vi "Handle Signal Density Plot.vi"(7 "State in":T1, 8 "error in (no error)":errorcluster, 10 "Alligned FFT Frame Out":refnum<class "2D Array f32.lvclass">, 11 "Signal Analysis in":refnum<class "Signal Analysis.lvclass">) -> (0 "error out":errorcluster, 2 "Signal Density Plot Available":bool, 3 "Signal Density Plot":refnum<class "2D Array f32.lvclass">, 5 "State out":T1)   [LabVIEW 2020, in "Signal Analysis.lvlib" / "Signal Analysis.lvclass"]
uses:
  Signal Analysis.lvclass
  <vilib>/Natan Biesmans/G2CPU GPU and CPU HPC Toolkit/G2CPU Libraries/Arrays/1DArray/u32/1D Array u32.lvclass
  <vilib>/Natan Biesmans/G2CPU GPU and CPU HPC Toolkit/G2CPU Libraries/Arrays/2DArray/s16/2D Array s16.lvclass
  <vilib>/Natan Biesmans/G2CPU GPU and CPU HPC Toolkit/G2CPU Libraries/Arrays/2DArray/f32/2D Array f32.lvclass
  C:/Program Files/National Instruments/LabVIEW 2025/vi.lib/Natan Biesmans/G2CPU GPU and CPU HPC Toolkit/G2CPU Libraries/Arrays/Array/Array Prototype.lvclass
  Signal Analysis.lvclass/Signal Analysis.ctl
  <vilib>/Natan Biesmans/G2CPU GPU and CPU HPC Toolkit/G2CPU Libraries/Arrays/1DArray/s32/1D Array s32.lvclass
  <vilib>/Natan Biesmans/G2CPU GPU and CPU HPC Toolkit/G2CPU Libraries/Arrays/1DArray/f32/1D Array f32.lvclass
  <vilib>/Natan Biesmans/G2CPU GPU and CPU HPC Toolkit/G2CPU Libraries/Arrays/Array/Array Prototype.lvclass
  <vilib>/Natan Biesmans/G2CPU GPU and CPU HPC Toolkit/G2CPU Libraries/Arrays/DataTypes/I32/s32.lvclass
  <vilib>/Natan Biesmans/G2CPU GPU and CPU HPC Toolkit/G2CPU Libraries/Arrays/1DArray/1D Array Prototype.lvclass
  <vilib>/Natan Biesmans/G2CPU GPU and CPU HPC Toolkit/G2CPU Libraries/Arrays/DataTypes/f32/f32.lvclass
  <vilib>/Natan Biesmans/G2CPU GPU and CPU HPC Toolkit/G2CPU Libraries/Arrays/2DArray/2D Array Prototype.lvclass
  C:/Program Files/National Instruments/LabVIEW 2025/vi.lib/Natan Biesmans/G2CPU GPU and CPU HPC Toolkit/G2CPU Libraries/Arrays/1DArray/1D Array Prototype.lvclass
  C:/Program Files/National Instruments/LabVIEW 2025/vi.lib/Natan Biesmans/G2CPU GPU and CPU HPC Toolkit/G2CPU Libraries/Arrays/1DArray/f32/1D Array f32.lvclass
  C:/Program Files/National Instruments/LabVIEW 2025/vi.lib/Natan Biesmans/G2CPU GPU and CPU HPC Toolkit/G2CPU Libraries/Arrays/DataTypes/f32/f32.lvclass
  d8d0d967-f4c4-454d-b5f2-45f85e871cba.vi
  Program Files/National Instruments/LabVIEW 2025/examples/Natan Biesmans/G2CPU GPU and CPU HPC Toolkit/_Examples/UI Acceleration/Signal Density Plot Config.ctl
  <vilib>/Natan Biesmans/G2CPU GPU and CPU HPC Toolkit/G2CPU Libraries/UI Acceleration/G2CPU Signal Density Plots.lvlib
  0e8233dc-15c9-41dc-9b30-8b63ab7c6b8c.vi
  c5ece696-53a1-4daa-a705-5cda5cc95be4.vi
  <vilib>/Utility/miscctls.llb/LVOffsetAndMultiplierTypeDef.ctl
  Helper Loop State.ctl
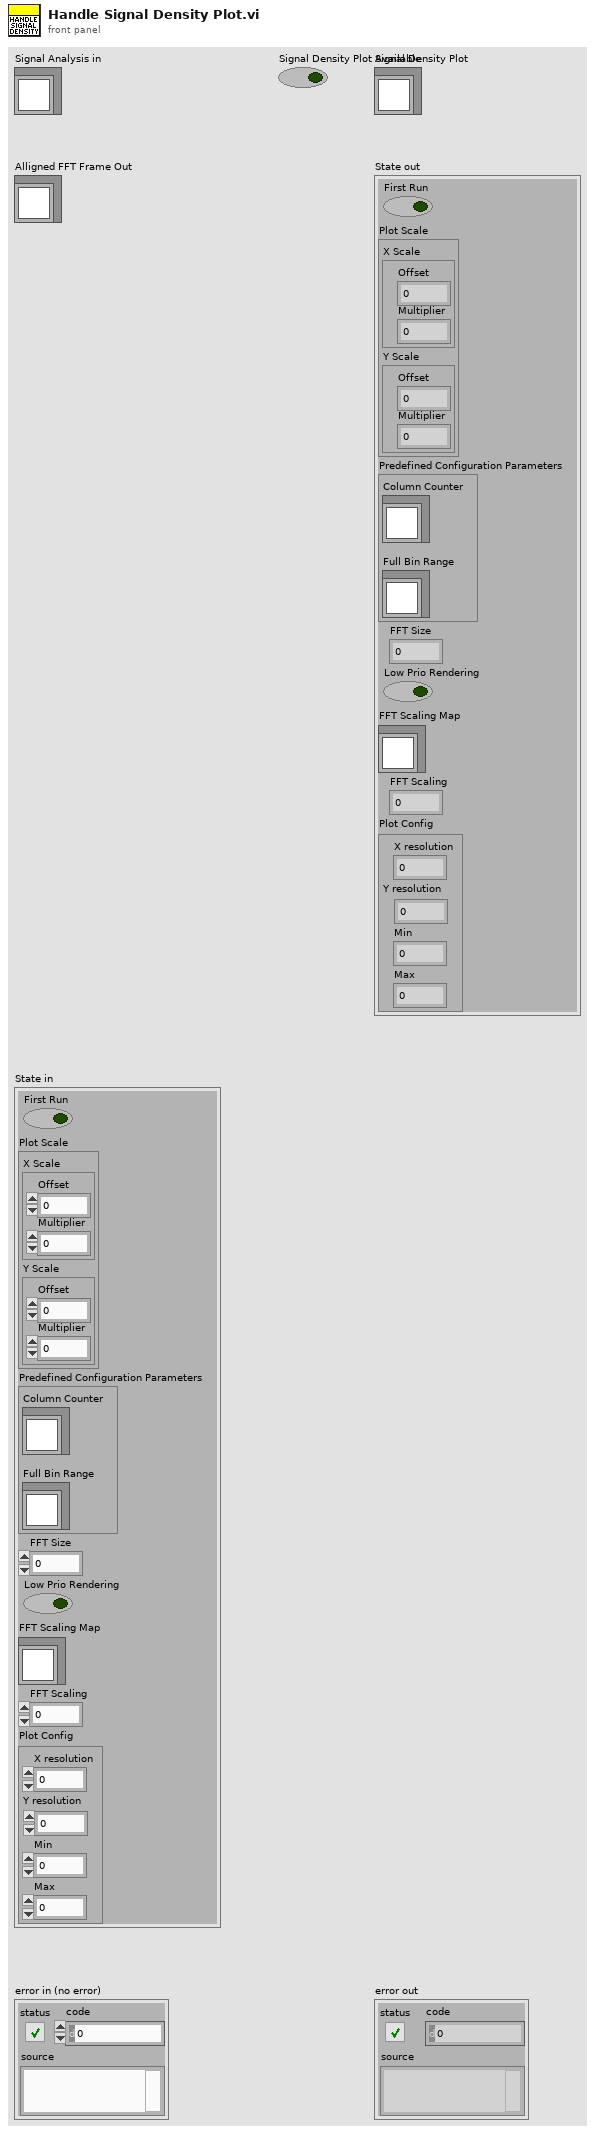
[diagram p1: front panel]
types:
  T1 = typedef "Signal Analysis.lvlib/Signal Analysis.lvclass/Helper Loop State.ctl" = cluster{"First Run":bool, "Plot Scale":cluster{"X Scale":T2, "Y Scale":T2}, "Predefined Configuration Parameters":cluster{"Column Counter":refnum<class "1D Array u32.lvclass">, "Full Bin Range":refnum<class "2D Array s16.lvclass">}, "FFT Size":i32, "Low Prio Rendering":bool, "FFT Scaling Map":refnum<class "1D Array u32.lvclass">, "FFT Scaling":dbl, "Graph Config":T3}
  T2 = typedef "LVOffsetAndMultiplierTypeDef.ctl" = cluster{"Offset":dbl, "Multiplier":dbl}
  T3 = typedef "G2CPU Signal Density Plots.lvlib/Signal Density Plot Config.ctl" = cluster{"X resolution":u64, "Y resolution":u64, "Min":sgl, "Max":sgl}
  T4 = cluster{"Column Counter":refnum<class "1D Array u32.lvclass">, "Full Bin Range":refnum<class "2D Array s16.lvclass">}
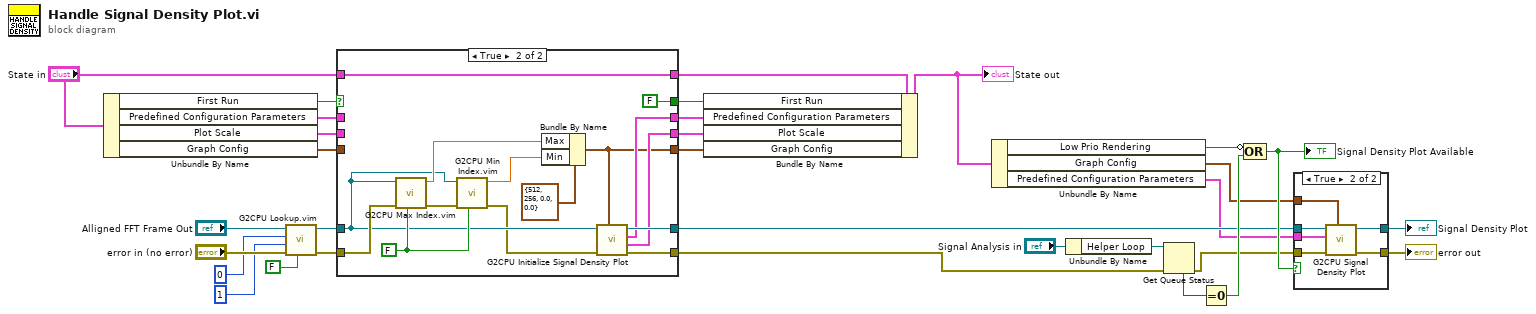
[diagram p0: block diagram]
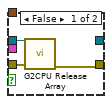
[diagram p3: hidden frame]
diagram:
  n1 = Unbundle By Name("State in") -> ("First Run"=w19:bool, "Predefined Configuration Parameters"=w20:T4, "Plot Scale"=w21:cluster{"X Scale":T2, "Y Scale":T2}, "Graph Config"=w29:T3)
  n2 = call "G2CPU Lookup.vim"("Auto Release Array In (Enabled)"=FALSE, "error in (no error)"="error in (no error)", "dim"=u64 1, "Indices (1D)"=0, "Array In"="Alligned FFT Frame Out") -> ("error out"=w31:errorcluster, "Indexed Array"=w8:refnum<class "1D Array f32.lvclass">)  [unwired: 5 in]
  n3 = case shown="True" w19 {
    selector: w19 -> [w38 _]
    tunnel: w8 -> [w37 w42]
    tunnel: [w37 w53] -> w10
    tunnel: [w32 w52] -> w14
    tunnel: [w35 w51] -> w23
    tunnel: [w36 w50] -> w2
    tunnel: [w38 FALSE] -> w22
    tunnel: w20 -> [w36 _]
    tunnel: w21 -> [w35 _]
    tunnel: "State in" -> [w34 w48]
    tunnel: [w34 w48] -> w24
    tunnel: w29 -> [w33 _]
    tunnel: [w33 w40] -> w4
    tunnel: w31 -> [w32 w43]
    frame False {
    }
    frame True {
      w44 = FALSE ("Auto Release (Enabled)")
      n4 = call "G2CPU Max Index.vim"("Auto Release (Enabled)"=w44, "error in (no error)"=w43, "Array First"=w42) -> ("error out"=w45:errorcluster, "real out"=w47:dbl)  [unwired: 5 in, 2 out]
      n5 = call "G2CPU Min Index.vim"("Auto Release (Enabled)"=w44, "error in (no error)"=w45, "Array First"=w42) -> ("error out"=w39:errorcluster, "real out"=w46:dbl)  [unwired: 5 in, 2 out]
      n6 = Bundle By Name(cluster=T3 {"X resolution"=512, "Y resolution"=256, "Min"=0.0, "Max"=0.0} ("Plot Config"), "Max"=w47, "Min"=w46) -> (w40:T3)
      n7 = call <vilib>:"G2CPU Initialize Signal Density Plot.vi"("Plot Config"=w40, "error in (no error)"=w39, "Data In"=w42) -> ("error out"=w52:errorcluster, "Plot Scale"=w51:cluster{"X Scale":T2, "Y Scale":T2}, "Predefined Configuration Parameters"=w50:T4, "Data Out (same as in)"=w53:refnum<class "1D Array f32.lvclass">)  [unwired: 5 in]
    }
  }
  n8 = Bundle By Name(cluster=w24, "First Run"=w22, "Predefined Configuration Parameters"=w2, "Plot Scale"=w23, "Graph Config"=w4) -> (w5:T1)
  "State out" <- w5
  n9 = Unbundle By Name(w5) -> ("Low Prio Rendering"=w25:bool, "Graph Config"=w3:T3, "Predefined Configuration Parameters"=w1:T4)
  n10 = Unbundle By Name("Signal Analysis in") -> ("Helper Loop"=w17:refnum<queue>)
  n11 = Get Queue Status(queue=w17, error in (no error)=w14) -> (error out=w15:errorcluster, # elements in queue=w18:i32)  [unwired: 1 in, 6 out]
  n12 = Equal To 0?(x=w18) -> (x = 0?=w26:bool)
  n13 = Compound Arithmetic op=OR(invert w25, w26) -> (w27:bool)
  "Signal Density Plot Available" <- w27
  n14 = case shown="True" w27 {
    tunnel: w10 -> [w55 w62]
    tunnel: w15 -> [w56 w61]
    tunnel: [w54 w60] -> w11
    tunnel: [_ w59] -> w12
    tunnel: w1 -> [_ w58]
    tunnel: w3 -> [_ w57]
    frame False {
      n15 = call <vilib>:"G2CPU Release Array.vi"("error in (no error)"=w56, "Array in"=w55) -> ("error out"=w54:errorcluster)  [unwired: 9 in]
    }
    frame True {
      n16 = call <vilib>:"G2CPU Signal Density Plot.vi"("Graph Config"=w57, "error in (no error)"=w61, "Predefined Configuration Parameters"=w58, "Data In"=w62) -> ("error out"=w60:errorcluster, "Signal Density Plot"=w59:refnum<class "2D Array f32.lvclass">)  [unwired: 6 in]
    }
  }
  "Signal Density Plot" <- w12
  "error out" <- w11
